vi "Select Buffer Elements.vi"(8 "error in (no error)":errorcluster, 10 "Item Indices":i32[](array[numeric]) step=1, 11 "DMM6500 in":refnum<class "DMM6500.lvclass">) -> (0 "error out":errorcluster, 2 "Selected Buffer Elements":string[](array[string]), 3 "DMM6500 out":refnum<class "DMM6500.lvclass">)   [LabVIEW 2023, in "HAF.lvlib" / "DMM6500.lvclass"]
uses:
  DMM6500.lvclass
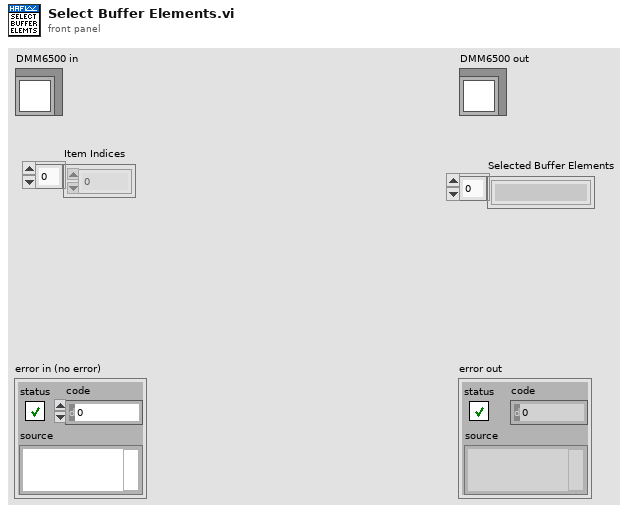
[diagram p1: front panel]
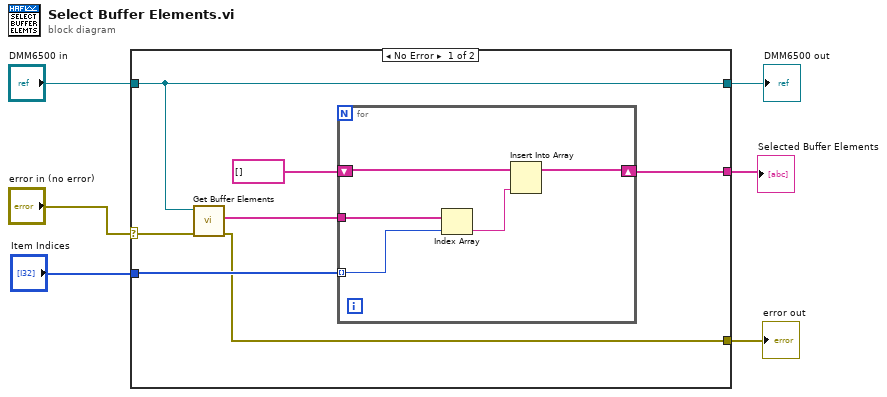
[diagram p0: block diagram]
diagram:
  n1 = case shown="No Error" "error in (no error)" {
    selector: "error in (no error)" -> [w13 w20]
    tunnel: [w7 w20] -> w5
    tunnel: [w8 w19] -> w3
    tunnel: "DMM6500 in" -> [w8 w19]
    tunnel: "Item Indices" -> [w10 _]
    tunnel: [w9 _] -> w1
    frame No Error {
      n2 = call "Get Buffer Elements.vi"("error in (no error)"=w13, "DMM6500 in"=w8) -> ("error out"=w7:errorcluster, "Buffer Elements"=w12:string[])  [unwired: 7 in, 1 out]
      n3 = for {
        tunnel: w12 -> [w18]
        shift-right: [w14] -> w9
        shift-left: string[] [] -> [w16]
        tunnel: w10 -> [w17] mode=indexing
        n4 = Index Array(array=w18, index=w17) -> (element=w15:string)
        n5 = Insert Into Array(array=w16, new element=w15) -> (w14:string[])  [unwired: 1 in]
      }
    }
    frame Error {
    }
  }
  "error out" <- w5
  "DMM6500 out" <- w3
  "Selected Buffer Elements" <- w1
